vi "QueryServer_GetTestDataTypesParameters.vi"(6 "error in (no error)":errorcluster, 9 "gRPCid":T3) -> (0 "error out":errorcluster, 2 "TestDataTypesParameters":T1, 3 "gRPCid out":T3)   [LabVIEW 2019, in "labview-grpc-query-server.lvlib"]
uses:
  labview-grpc-query-server.lvlib
  VIs/grpcId.ctl
  QueryServer_TestDataTypesParameters.ctl
  QueryServer_DataTypeTest.ctl
  ea7aee44-32c1-4253-ac5d-59c6ef46377d.vi
  VIs/gprc-support.lvlib
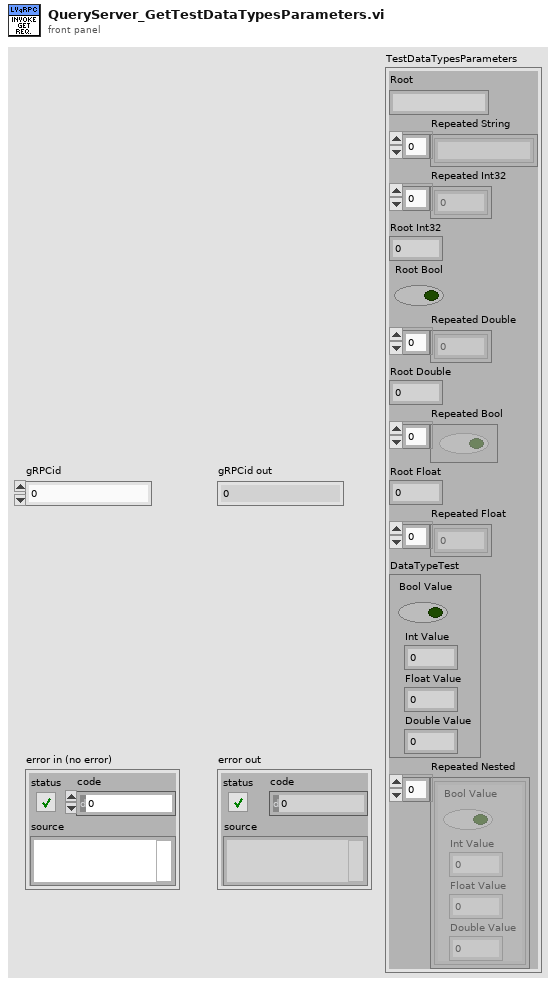
[diagram p1: front panel]
types:
  T1 = typedef "labview-grpc-query-server.lvlib/QueryServer_TestDataTypesParameters.ctl" = cluster{"Root":string, "Repeated String":string[], "Repeated Int32":i32[], "Root Int32":i32, "Root Bool":bool, "Repeated Double":dbl[], "Root Double":dbl, "Repeated Bool":bool[], "Root Float":sgl, "Repeated Float":sgl[], "DataTypeTest":T2, "Repeated Nested":T2[]}
  T2 = typedef "labview-grpc-query-server.lvlib/QueryServer_DataTypeTest.ctl" = cluster{"Bool Value":bool, "Int Value":i32, "Float Value":sgl, "Double Value":dbl}
  T3 = typedef "gprc-support.lvlib/grpcId.ctl" = u64
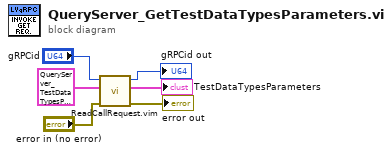
[diagram p0: block diagram]
diagram:
  n1 = call "ReadCallRequest.vim"("error in (no error)"="error in (no error)", "Data Type"=T1 {"Root"="", "Repeated String"=[], "Repeated Int32"=[], "Root Int32"=42, "Root Bool"=TRUE, "Repeated Double"=[67.8], "Root Double"=42.42, "Repeated Bool"=[], "Root Float"=0.0, "Repeated Float"=[], "DataTypeTest"={"Bool Value"=FALSE, "Int Value"=0, "Float Value"=0.0, "Double Value"=0.0}, "Repeated Nested"=[]} ("TestDataTypesParameters"), "gRPCid in"="gRPCid") -> ("error out"=→"error out":errorcluster, "Request Data"=→"TestDataTypesParameters":T1, "gRPCid out"=→"gRPCid out":T3)  [unwired: 6 in]
